vi "SetPort.vi"(8 "error in (no error)":errorcluster, 9 "Value":u8, 10 "Port":u8, 11 "Simulated Device in":refnum<class "Simulated Device.lvclass">) -> (0 "error out":errorcluster, 3 "Simulated Device out":refnum<class "Simulated Device.lvclass">)   [LabVIEW 2020, in "Simulated Device.lvclass"]
doc: "Set a value on a port on the target device."
uses:
  Simulated Device.lvclass
  Controls/Device Command Code.ctl
  Controls/Device Code.ctl
  <vilib>/Utility/error.llb/Error Cluster From Error Code.vi
  <vilib>/ErrorRing/Error Ring.xnode
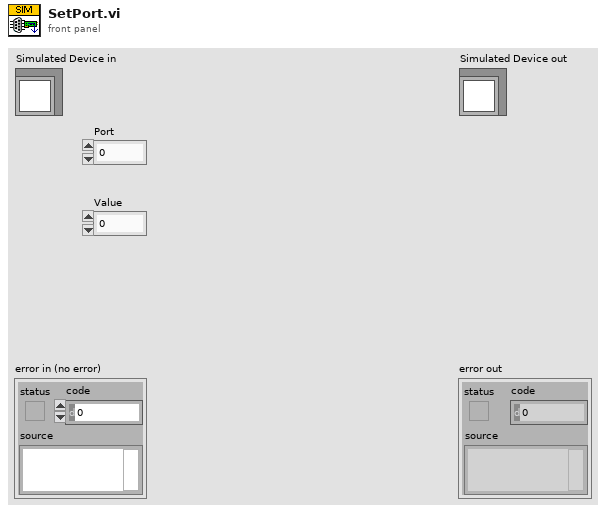
[diagram p1: front panel]
types:
  T1 = typedef "Device Code.ctl" = string
  T2 = typedef "Device Command Code.ctl" = string
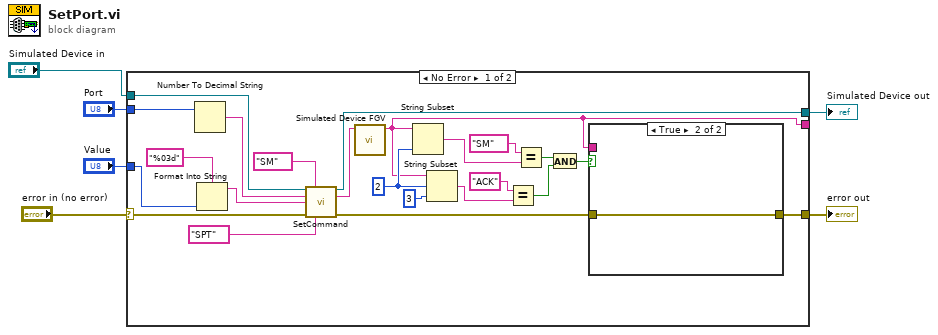
[diagram p0: block diagram]
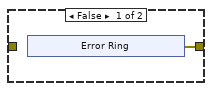
[diagram p2: hidden frame]
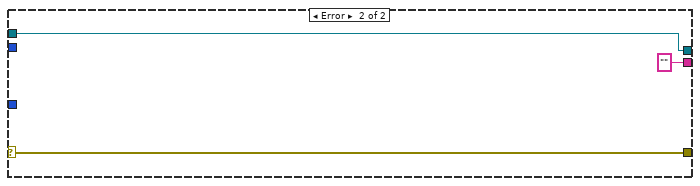
[diagram p3: hidden frame]
diagram:
  n1 = case shown="No Error" "error in (no error)" {
    selector: "error in (no error)" -> [w29 w39]
    tunnel: [w18 w39] -> w4
    tunnel: [w24 w37] -> w5
    tunnel: "Port" -> [w26 _]
    tunnel: [w7 "" ("read buffer")] -> _
    tunnel: "Value" -> [w11 _]
    tunnel: "Simulated Device in" -> [w12 w37]
    frame No Error {
      w22 = 2 ("length (rest)")
      n2 = Number To Decimal String(number=w26) -> (decimal integer string=w25:string)  [unwired: 1 in]
      n3 = Format Into String(format string="%03d", w11) -> (resulting string=w10:string)  [unwired: 2 in, 1 out]
      n4 = call-dynamic "SetCommand.vi"("Simulated Device in"=w12, "Device Code"=T1 "SM", "Parameter 1"=w25, "Parameter 2"=w10, "error in (no error)"=w29, "Command Code"=T2 "SPT") -> ("Simulated Device out"=w24:refnum<class "Simulated Device.lvclass">, "Command"=w8:string, "error out"=w14:errorcluster)  [unwired: 7 in]
      n5 = call "Simulated Device FGV.vi"("Request"=w8) -> ("Response"=w7:string)  [unwired: 10 in]
      n6 = String Subset(string=w7, length (rest)=w22) -> (substring=w16:string)  [unwired: 1 in]
      n7 = String Subset(string=w7, offset (0)=w22, length (rest)=3 ("length (rest)")) -> (substring=w23:string)
      n8 = Equal?(x="ACK", y=w23) -> (x = y?=w20:bool)
      n9 = Equal?(x=T1 "SM" ("Device Code"), y=w16) -> (x = y?=w17:bool)
      n10 = And(x=w17, y=w20) -> (x .and. y?=w19:bool)
      n11 = case shown="True" w19 {
        tunnel: w14 -> [_ w36]
        tunnel: [w30 w36] -> w18
        tunnel: w7 -> [_ _]
        frame False {
          n12 = xnode "Error Ring"() -> ("error out"=w30:errorcluster)
        }
        frame True {
        }
      }
    }
    frame Error {
    }
  }
  "error out" <- w4
  "Simulated Device out" <- w5
